vi "test Ntrip-Client command.vi"() -> ()   [LabVIEW 2019]
panel:
  in  "Ntrip client info":T1={"id"="GET /YONS-RTCM32-M5 HTTP/1.0\r\nUser-Agent: NTRIP YbbaekRLmodelNTRIPClient/20210614\r\nAccept: */*\r\nConnection: close\n\rAuthorization: Basic c2VvdWw6c2VvdWw=\r\n\r\n", "pwd"="GET /YONS-RTCM32-M5 HTTP/1.0\r\nUser-Agent: NTRIP YbbaekRLmodelNTRIPClient/20210614\r\nAccept: */*\r\nConnection: close\n\rAuthorization: Basic c2VvdWw6c2VvdWw=\r\n\r\n", "ref pt name"="GET /YONS-RTCM32-M5 HTTP/1.0\r\nUser-Agent: NTRIP YbbaekRLmodelNTRIPClient/20210614\r\nAccept: */*\r\nConnection: close\n\rAuthorization: Basic c2VvdWw6c2VvdWw=\r\n\r\n"}
  out "concatenated string":string
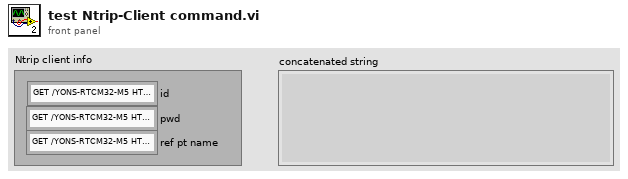
[diagram p1: front panel]
types:
  T1 = cluster{"id":string, "pwd":string, "ref pt name":string}
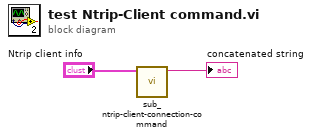
[diagram p0: block diagram]
diagram:
  n1 = call "sub_ntrip-client-connection-command.vi"("Ntrip client info"="Ntrip client info") -> ("String"=→"concatenated string":string)  [unwired: 10 in]
